vi "Write AO.vi"(8 "error in (no error)":errorcluster, 10 "AO":cluster{"output config":T1, "output signal":T2}, 11 "lockin in":refnum<class "lockin.lvclass">) -> (0 "error out":errorcluster, 3 "lockin out":refnum<class "lockin.lvclass">)   [LabVIEW 2016, in "lockin.lvclass"]
uses:
  lockin.lvclass
  Typedefs/lockin_output_configuration.ctl
  Typedefs/lockin_output_signals.ctl
  lockin.lvclass/lockin.ctl
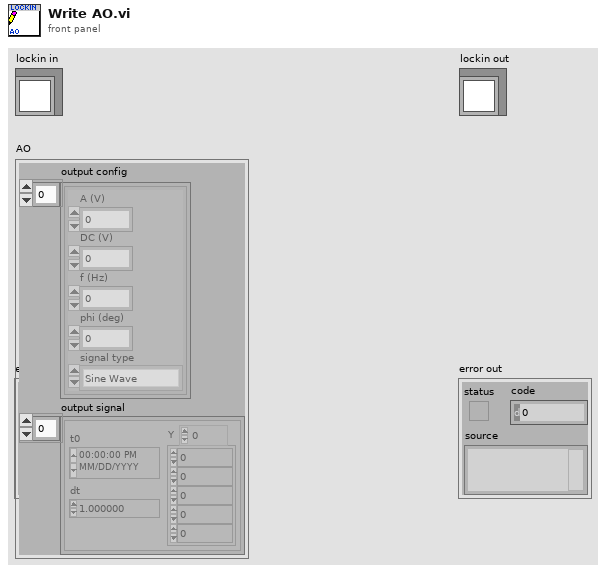
[diagram p1: front panel]
types:
  T1 = typedef "lockin.lvclass/lockin_output_configuration.ctl" = cluster{"A (V)":dbl, "DC (V)":dbl, "f (Hz)":dbl, "phi (deg)":dbl, "signal type":enum16{"Sine Wave", "Triangle Wave", "Square Wave", "Sawtooth Wave"}}[]
  T2 = typedef "lockin.lvclass/lockin_output_signals.ctl" = waveform(dbl)[]
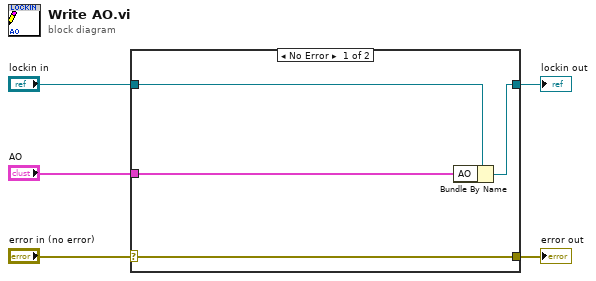
[diagram p0: block diagram]
diagram:
  n1 = case shown="No Error" "error in (no error)" {
    selector: "error in (no error)" -> [w9 w10]
    tunnel: [w9 w10] -> w4
    tunnel: [w7 w11] -> w2
    tunnel: "lockin in" -> [w8 w11]
    tunnel: "AO" -> [w6 _]
    frame No Error {
      n2 = Bundle By Name(cluster=w8, "AO"=w6) -> (w7:refnum<class "lockin.lvclass">)
    }
    frame Error {
    }
  }
  "error out" <- w4
  "lockin out" <- w2
